vi "oa_Compute Waterfall Plot Grid Lines.vi"(4 "zoom factor":dbl=5.0, 5 "Y range":cluster{"min":dbl, "max":dbl}={"min"=5.0, "max"=5.0} {"max" format="%.6f"; "min" format="%.6f"}, 6 "Y scale":cluster{"offset":dbl, "multiplier":dbl} {"multiplier" format="%.2f"; "offset" format="%.2f"}, 7 "X scale":cluster{"offset":dbl, "multiplier":dbl} {"multiplier" format="%.2f"; "offset" format="%.2f"}, 8 "max x axis offset":dbl, 9 "# of bins":i32, 10 "grid lines to plot [Hz/Order]":dbl[](array[numeric]), 11 "waterfall plot":cluster{"X0":dbl, "dX":dbl, "Y":dbl[]}[](array[cluster]) {"Y" format="%.2f"; "dX" format="%.2f"; "X0" format="%.2f"}) -> (0 "# of axis lines":i32, 1 "# of grid lines":i32, 3 "waterfall plot out":cluster{"X0":dbl, "dX":dbl, "Y":dbl[]}[](array[cluster]) {"Y" format="%.2f"; "dX" format="%.2f"; "X0" format="%.2f"})   [LabVIEW 2017]
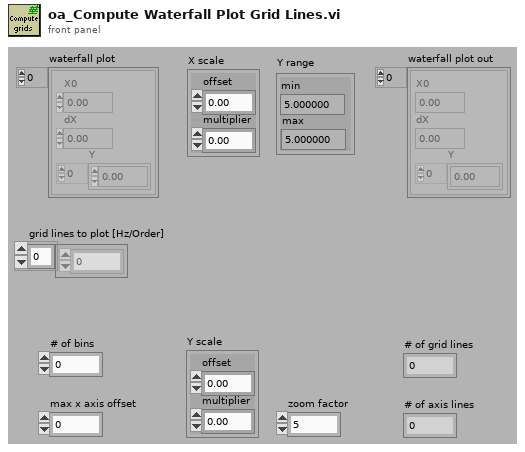
[diagram p1: front panel]
types:
  T1 = cluster{"Numeric":dbl, "max x axis offset":dbl, dbl[]}
  T2 = cluster{"offset":dbl, "max x axis offset":dbl, dbl[]}
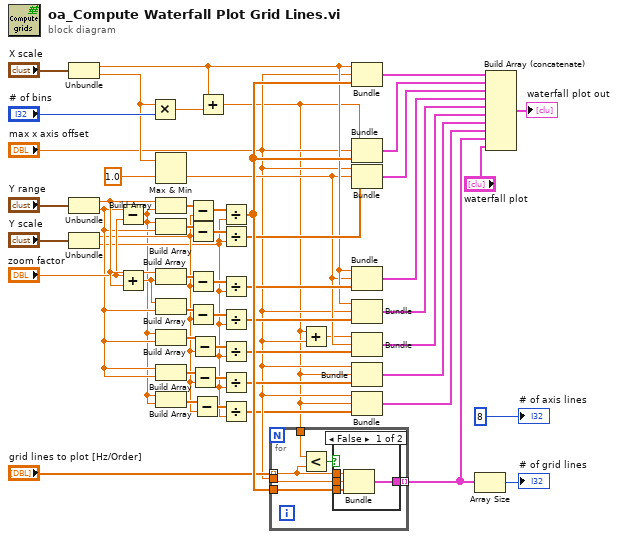
[diagram p0: block diagram]
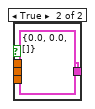
[diagram p2: hidden frame]
diagram:
  n1 = Unbundle("X scale") -> ("offset"=w21:dbl, "multiplier"=w27:dbl)
  n2 = Unbundle("Y range") -> ("min"=w14:dbl, "max"=w12:dbl)
  n3 = Unbundle("Y scale") -> ("offset"=w8:dbl, "multiplier"=w7:dbl)
  n4 = Subtract(x=w12, y="zoom factor") -> (x-y=w4:dbl)
  n5 = Add(x="zoom factor", y=w14) -> (x+y=w18:dbl)
  n6 = Multiply(x=w27, y="# of bins") -> (x*y=w25:dbl)
  n7 = Max & Min(x=w27, y=1.0) -> (min(x,y)=w20:dbl)  [unwired: 1 out]
  n8 = Build Array(w14, w4) -> (w44:dbl[])
  n9 = Build Array(w4, w12) -> (w41:dbl[])
  n10 = Build Array(w14, w18) -> (w36:dbl[])
  n11 = Build Array(w18, w12) -> (w31:dbl[])
  n12 = Build Array(w4, w12) -> (w16:dbl[])
  n13 = Build Array(w12, w12) -> (w23:dbl[])
  n14 = Build Array(w4, w4) -> (w9:dbl[])
  n15 = Subtract(x=w44, y=w8) -> (x-y=w43:dbl[])
  n16 = Subtract(x=w41, y=w8) -> (x-y=w40:dbl[])
  n17 = Subtract(x=w36, y=w8) -> (x-y=w37:dbl[])
  n18 = Subtract(x=w31, y=w8) -> (x-y=w32:dbl[])
  n19 = Subtract(x=w16, y=w8) -> (x-y=w17:dbl[])
  n20 = Subtract(x=w23, y=w8) -> (x-y=w24:dbl[])
  n21 = Subtract(x=w9, y=w8) -> (x-y=w10:dbl[])
  n22 = Add(x=w21, y=w25) -> (x+y=w1:dbl)
  n23 = Divide(x=w43, y=w7) -> (x/y=w42:dbl[])
  n24 = Divide(x=w40, y=w7) -> (x/y=w39:dbl[])
  n25 = Divide(x=w37, y=w7) -> (x/y=w35:dbl[])
  n26 = Divide(x=w32, y=w7) -> (x/y=w29:dbl[])
  n27 = Divide(x=w17, y=w7) -> (x/y=w15:dbl[])
  n28 = Divide(x=w24, y=w7) -> (x/y=w22:dbl[])
  n29 = Divide(x=w10, y=w7) -> (x/y=w6:dbl[])
  n30 = for {
    tunnel: "grid lines to plot [Hz/Order]" -> [w56] mode=indexing
    tunnel: "max x axis offset" -> [w58]
    tunnel: w42 -> [w60]
    tunnel: [w59] -> w2 mode=indexing
    tunnel: w1 -> [w57]
    n31 = Less?(x=w57, y=w56) -> (x < y?=w55:bool)
    n32 = case shown="False" w55 {
      tunnel: w60 -> [w64 _]
      tunnel: [w63 T1 {"Numeric"=0.0, "max x axis offset"=0.0, []}] -> w59
      tunnel: w58 -> [w62 _]
      tunnel: w56 -> [w61 _]
      frame False {
        n33 = Bundle("Numeric"=w61, "max x axis offset"=w62, w64) -> (w63:T1)  [unwired: 1 in]
      }
      frame True {
      }
    }
  }
  n34 = Add(x=w1, y="max x axis offset") -> (x+y=w19:dbl)
  n35 = Bundle("offset"=w21, "max x axis offset"="max x axis offset", w42) -> (w52:T2)  [unwired: 1 in]
  n36 = Bundle(w1, "max x axis offset"="max x axis offset", w42) -> (w49:cluster{dbl, "max x axis offset":dbl, dbl[]})  [unwired: 1 in]
  n37 = Bundle("max x axis offset"="max x axis offset", w20, w39) -> (w48:cluster{"max x axis offset":dbl, dbl, dbl[]})  [unwired: 1 in]
  n38 = Bundle("offset"=w21, w20, w35) -> (w33:cluster{"offset":dbl, dbl, dbl[]})  [unwired: 1 in]
  n39 = Bundle("offset"=w21, "max x axis offset"="max x axis offset", w29) -> (w30:T2)  [unwired: 1 in]
  n40 = Bundle(w19, w20, w15) -> (w28:cluster{dbl, dbl, dbl[]})  [unwired: 1 in]
  n41 = Bundle("max x axis offset"="max x axis offset", w1, w22) -> (w26:cluster{"max x axis offset":dbl, dbl, dbl[]})  [unwired: 1 in]
  n42 = Bundle("max x axis offset"="max x axis offset", w1, w6) -> (w5:cluster{"max x axis offset":dbl, dbl, dbl[]})  [unwired: 1 in]
  n43 = Array Size(array=w2) -> (size(s)=→"# of grid lines":i32)
  n44 = Build Array (concatenate)(w52, w49, w48, w33, w30, w28, w26, w5, w2, "waterfall plot") -> (→"waterfall plot out":cluster{"X0":dbl, "dX":dbl, "Y":dbl[]}[])
  "# of axis lines" <- 8 ("# of axis lines")
